vi "UTILITY Get Point File List.vi"(8 "error in (no error)":errorcluster, 11 "Folder Path":path) -> (0 "error out":errorcluster, 3 "Point File Names":string[](array[string]))   [LabVIEW 2016]
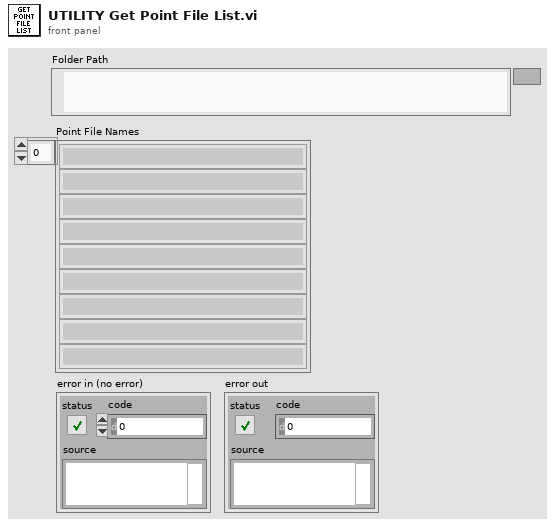
[diagram p1: front panel]
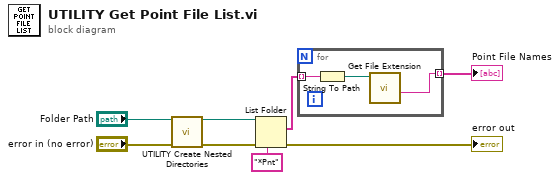
[diagram p0: block diagram]
diagram:
  n1 = call "UTILITY Create Nested Directories.vi"("path to create"="Folder Path", "error in"="error in (no error)") -> ("created path"=w2:path, "error out"=w1:errorcluster)  [unwired: 11 in, 1 out]
  n2 = List Folder(path=w2, pattern="*Pnt", error in=w1) -> (filenames=w7:string[], error out=→"error out":errorcluster)  [unwired: 1 in, 2 out]
  n3 = for {
    tunnel: w7 -> [w10] mode=indexing
    tunnel: [w9] -> w8 mode=indexing
    n4 = String To Path(string=w10) -> (path=w11:path)
    n5 = call <vilib>:"Get File Extension.vi"("file"=w11) -> ("filename without extension"=w9:string)  [unwired: 6 in, 4 out]
  }
  "Point File Names" <- w8
